vi "CvrtCell2Data.vi"(8 "error in (no error)":errorcluster, 9 "ge_HdrNames":T1, 10 "Item Name":string, 11 "Tachometer in":refnum<class "Tachometer.lvclass">) -> (0 "error out":errorcluster, 3 "Tachometer out":refnum<class "Tachometer.lvclass">)   [LabVIEW 2012, in "Measurement Channels.lvlib" / "Tachometer.lvclass"]
uses:
  Tachometer.lvclass
  Common/Controls/HeaderNames.ctl
  Tachometer.lvclass/Tachometer.ctl
  Class Frequency/Frequency.lvclass
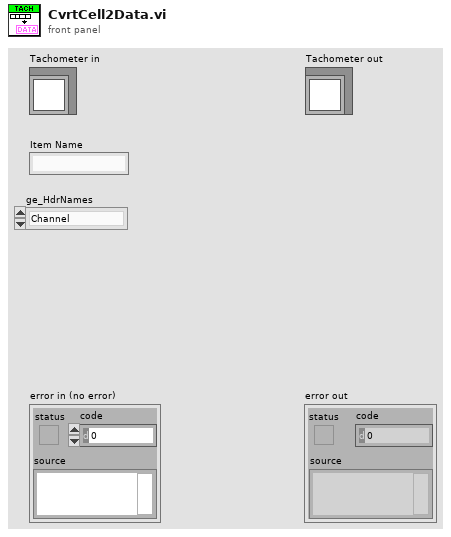
[diagram p1: front panel]
types:
  T1 = typedef "HeaderNames.ctl" = enum16{"Channel", "Device", "Spacer", "Description", "MB", "Range", "Terminal", "Coupling", "Thresh (V)", "Pulse/Rev", "Slope", "Min EU", "Min RPM", "mV/EU", "Iex", "Temp Units", "Type", "CJC Src", "CJC Val", "Ro", "Wire Cfg", "Strain Mode", "Vex", "Bridge Type", "GF", "Gauge Res", "Poisson", "Lead Res", "Init Strain", "GAF", "Scale", "Offset", "Unit (EU)", "dB?", "dB Ref", "Cal Mag", "Cal Units", "Max Temp", "Min Temp", "Max Strain", "Min Strain"}
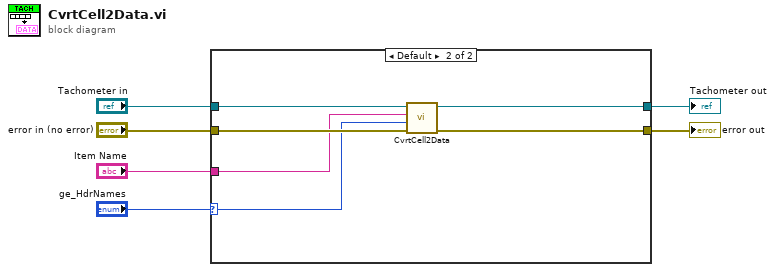
[diagram p0: block diagram]
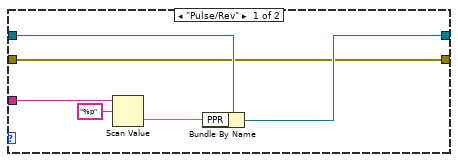
[diagram p2: hidden frame]
diagram:
  n1 = case shown="Default" "ge_HdrNames" {
    selector: "ge_HdrNames" -> [_ w13]
    tunnel: "Tachometer in" -> [w12 w18]
    tunnel: [w11 w17] -> w5
    tunnel: "error in (no error)" -> [w10 w16]
    tunnel: [w10 w15] -> w3
    tunnel: "Item Name" -> [w8 w14]
    frame "Pulse/Rev" {
      n2 = Scan Value(string=w8, format string="%p") -> (value=w7:dbl)  [unwired: 1 in, 1 out]
      n3 = Bundle By Name(cluster=w12, "PPR"=w7) -> (w11:refnum<class "Tachometer.lvclass">)
    }
    frame Default {
      n4 = call-parent "CvrtCell2Data.vi"("error in (no error)"=w16, "ge_HdrNames"=w13, "Item Name"=w14, "Frequency in"=w18) -> ("error out"=w15:errorcluster, "Frequency out"=w17:refnum<class "Tachometer.lvclass">)  [unwired: 6 in]
    }
  }
  "error out" <- w3
  "Tachometer out" <- w5
